vi "Fibonacci Sequence Custom Test.vi"(3 "Error In":errorcluster, 4 "Solution VI":path, 5 "User VI":path) -> (0 "Error Out":errorcluster, 2 "Results":T1={"Id"="", "Score"={"Status"=enum."Passed", "cpu_time"=-1, "max_memory"=-1, "style_score"=-1, "score0"="", "score1"="", "score2"="", "score3"="", "score4"="", "score5"=""}})   [LabVIEW 2013]
doc: "This VI is a template for a custom users test. The User VI control will provide the absolute path to the VI to test. The solution VI control will provide the absolute path to the solution VI. The Results indicator should be populated with the results from testing the user submitted VI."
uses:
  <vilib>/LabVIEW Hacker/VIChallenge/Private/Grader/Type Defs/Grader Result.ctl
  <vilib>/LabVIEW Hacker/VIChallenge/Private/Type Defs/Database/Score.ctl
  <vilib>/LabVIEW Hacker/VIChallenge/Private/Grader/Type Defs/UTF Status.ctl
  <vilib>/LabVIEW Hacker/VIChallenge/VIChallenge.lvlib
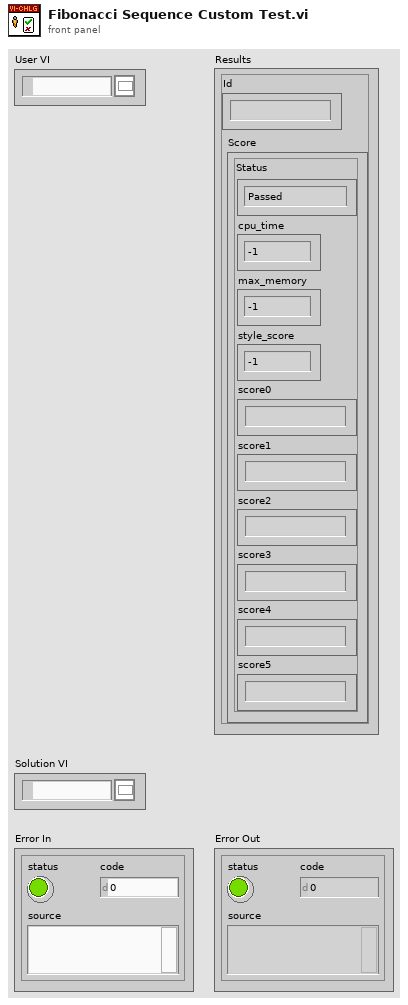
[diagram p1: front panel]
types:
  T1 = typedef "VIChallenge.lvlib/Grader Result.ctl" = cluster{"Id":string, "Score":T2}
  T2 = typedef "VIChallenge.lvlib/Score.ctl" = cluster{"Status":T3, "cpu_time":i32, "max_memory":i32, "style_score":i32, "score0":string, "score1":string, "score2":string, "score3":string, "score4":string, "score5":string}
  T3 = typedef "VIChallenge.lvlib/UTF Status.ctl" = enum16{"Null", "Passed", "Failed", "Error", "Skipped", "Not Processed"}
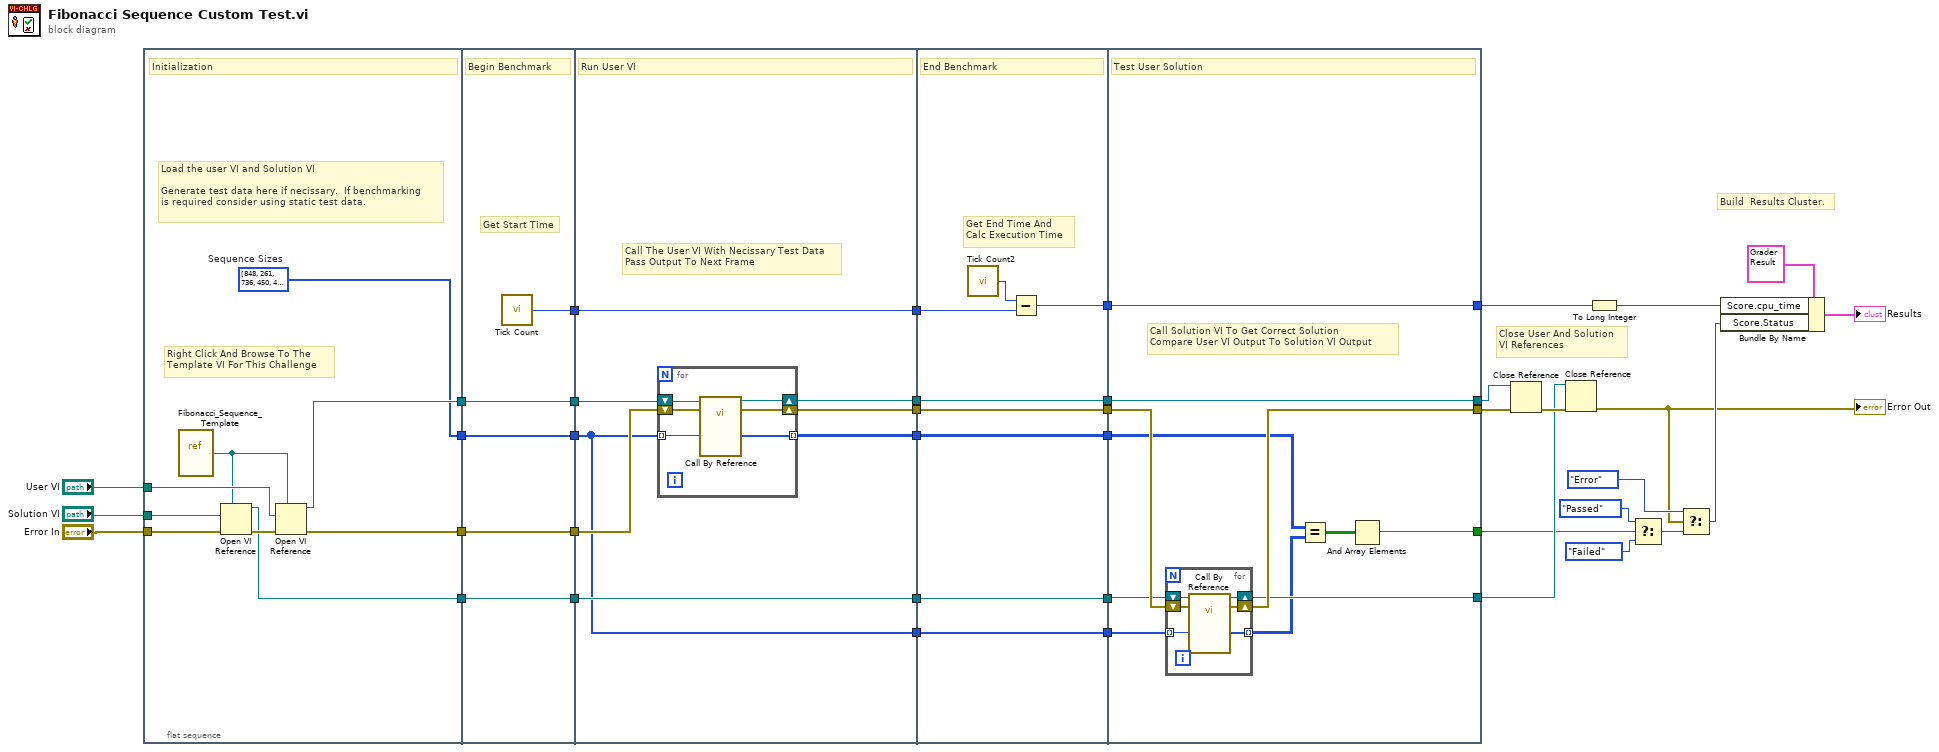
[diagram p0: block diagram]
diagram:
  # "Build  Results Cluster."
  # "Close User And Solution\nVI References"
  n1 = flat-sequence {
    tunnel: "User VI" -> [w48]
    tunnel: "Solution VI" -> [w47]
    tunnel: "Error In" -> [w45]
    tunnel: [w43] -> w36
    tunnel: [w42] -> w33
    tunnel: [w41] -> w31
    tunnel: [w40] -> w5
    tunnel: w36 -> [w53]
    tunnel: [w53] -> w35
    tunnel: [w52] -> w34
    tunnel: w33 -> [w52]
    tunnel: [w51] -> w32
    tunnel: w31 -> [w51]
    tunnel: [w50] -> w28
    tunnel: [w49] -> w6
    tunnel: w5 -> [w49]
    tunnel: w35 -> [w61]
    tunnel: w34 -> [w56]
    tunnel: w32 -> [w58]
    tunnel: [w60] -> w30
    tunnel: [w59] -> w29
    tunnel: w28 -> [w59]
    tunnel: [w58] -> w27
    tunnel: [w57] -> w24
    tunnel: w6 -> [w54]
    tunnel: [w55] -> w4
    tunnel: [w54] -> w2
    tunnel: w30 -> [w75]
    tunnel: w29 -> [w73]
    tunnel: w27 -> [w71]
    tunnel: [w75] -> w26
    tunnel: [w72] -> w25
    tunnel: w24 -> [w72]
    tunnel: [w71] -> w23
    tunnel: [w70] -> w16
    tunnel: w4 -> [w69]
    tunnel: [w69] -> w3
    tunnel: w2 -> [w68]
    tunnel: [w68] -> w1
    tunnel: w26 -> [w86]
    tunnel: [w85] -> w21
    tunnel: w25 -> [w84]
    tunnel: w23 -> [w81]
    tunnel: [w84] -> w22
    tunnel: [w83] -> w19
    tunnel: [w77] -> w10
    tunnel: [w82] -> w8
    tunnel: w16 -> [w82]
    tunnel: w3 -> [w79]
    tunnel: w1 -> [w76]
    frame #0 {
      w40 = i32[] [848, 261, 736, 450, 49, 224, 115, 680, 362, 624, 388, 820, 380, 134, 918, 80, 325, 741, 294, 696, 691, 389, 915, 94, 83, 534, 690, 884, 357, 231, 350, 306, 397, 577, 143, 331, 674, 651, 1, 955, 283, 492, 300, 331, 708, 110, 471, 604, 662, 688, 974, 81, 248, 860, 939, 728, 688, 739, 914, 177, 478, 553, 362, 47, 974, 305, 23, 21, 961, 618, 48, 320, 824, 858, 708, 83, 455, 633, 566, 303, 59, 686, 446, 422, 553, 816, 890, 2, 124, 380, 763, 747, 589, 93, 187, 708, 580, 173, 140, 759, 875, 436, 81, 583, 744, 843, 55, 23, 506, 335, 786, 137, 961, 736, 735, 404, 389, 322, 516, 500, 871, 607, 169, 214, 714, 459, 981, 620, 127, 889, 996, 708, 646, 29, 17, 401, 67, 538, 594, 639, 844, 321, 534, 599, 949, 132, 959, 525, 926, 960, 244, 913, 765, 714, 731, 554, 404, 451, 552, 639, 884, 506, 368, 394, 643, 586, 679, 689, 152, 774, 886, 928, 397, 633, 717, 929, 746, 21, 458, 364, 305, 218, 804, 475, 133, 567, 281, 12, 347, 932, 314, 835, 578, 181, 993, 288, 712, 262, 260, 91, 964, 436, 327, 78, 878, 660, 65, 334, 547, 455, 778, 594, 121, 44, 489, 594, 881, 98, 813, 344, 90, 360, 406, 840, 774, 262, 998, 166, 46, 997, 788, 862, 536, 417, 925, 762, 322, 598, 370, 909, 748, 627, 584, 320, 282, 604, 44, 710, 497, 951, 335, 283, 91, 467, 946, 286, 489, 482, 87, 572, 862, 986, 787, 68, 195, 928, 903, 904, 126, 315, 95, 514, 475, 508, 853, 889, 676, 678, 847, 157, 343, 368, 75, 163, 836, 3, 966, 743, 798, 794, 237, 376, 413, 65, 582, 245, 774, 480, 829, 614, 686, 122, 514, 932, 846, 794, 954, 919, 415, 973, 23, 812, 378, 892, 469, 770, 425, 619, 816, 806, 624, 930, 396, 924, 740, 375, 364, 624, 699, 2, 185, 252, 89, 251, 824, 889, 358, 576, 761, 308, 923, 706, 486, 608, 91, 184, 203, 396, 828, 131, 551, 331, 927, 347, 107, 109, 761, 87, 604, 488, 493, 846, 311, 631, 718, 289, 455, 96, 6, 201, 112, 115, 41, 144, 712, 178, 234, 10, 243, 314, 219, 630, 933, 189, 994, 272, 630, 689, 786, 645, 666, 962, 473, 347, 638, 288, 419, 479, 61, 892, 642, 116, 159, 121, 959, 127, 689, 78, 442, 139, 225, 401, 885, 423, 301, 523, 728, 503, 196, 240, 706, 88, 328, 817, 945, 290, 424, 898, 100, 923, 563, 494, 988, 623, 397, 721, 670, 5, 211, 665, 13, 983, 56, 546, 475, 834, 15, 267, 949, 679, 62, 883, 726, 338, 746, 647, 180, 663, 225, 811, 859, 193, 194, 622, 754, 36, 699, 553, 75, 272, 335, 411, 549, 283, 118, 596, 976, 703, 441, 757, 926, 643, 756, 972, 890, 809, 436, 888, 959, 628, 728, 440, 109, 936, 547, 85, 481, 662, 473, 998, 142, 523, 970, 102, 646, 409, 813, 527, 60, 964, 731, 626, 129, 447, 710, 341, 910, 783, 339, 323, 585, 789, 799, 348, 594, 900, 60, 187, 501, 465, 62, 342, 299, 766, 881, 852, 242, 797, 750, 195, 47, 147, 305, 346, 164, 729, 603, 95, 221, 599, 936, 835, 98, 563, 343, 600, 448, 901, 261, 506, 895, 123, 618, 247, 723, 111, 33, 622, 791, 146, 844, 893, 264, 193, 140, 812, 415, 964, 139, 451, 646, 421, 102, 219, 841, 462, 558, 685, 158, 566, 78, 620, 638, 871, 637, 255, 838, 673, 432, 706, 240, 394, 919, 183, 151, 623, 472, 154, 598, 386, 985, 310, 44, 434, 942, 798, 128, 603, 262, 830, 412, 468, 638, 461, 970, 391, 78, 305, 91, 931, 936, 536, 401, 833, 166, 652, 115, 107, 146, 662, 259, 508, 298, 100, 895, 783, 482, 689, 71, 542, 324, 325, 967, 615, 582, 917, 651, 753, 575, 395, 517, 391, 912, 482, 970, 847, 337, 148, 567, 853, 763, 815, 510, 317, 576, 546, 385, 843, 683, 614, 828, 683, 350, 881, 604, 470, 521, 834, 619, 198, 719, 493, 870, 299, 89, 868, 360, 825, 583, 845, 636, 800, 387, 697, 277, 41, 108, 542, 250, 72, 772, 558, 586, 116, 253, 576, 407, 9, 762, 737, 551, 902, 595, 757, 422, 749, 63, 247, 6, 860, 221, 691, 199, 470, 459, 119, 202, 214, 626, 574, 99, 331, 231, 838, 933, 251, 629, 643, 57, 200, 368, 858, 551, 181, 308, 428, 654, 482, 434, 209, 189, 824, 611, 981, 166, 259, 750, 298, 415, 582, 736, 14, 783, 840, 240, 999, 364, 850, 15, 108, 561, 200, 33, 736, 873, 429, 990, 447, 583, 935, 617, 989, 242, 693, 950, 379, 859, 740, 503, 546, 586, 837, 172, 264, 709, 711, 159, 187, 136, 633, 432, 985, 157, 144, 839, 491, 746, 741, 457, 318, 386, 456, 129, 64, 661, 262, 409, 472, 577, 720, 610, 99, 166, 181, 952, 359, 128, 375, 239, 811, 732, 260, 576, 57, 173, 334, 611, 583, 171, 388, 318, 462, 594, 27, 662, 567, 844, 850, 847, 301, 486, 99, 579, 296, 865, 713, 153, 480, 724, 632, 613, 807, 88, 963, 833, 129, 314, 592, 102, 368, 541, 329, 39, 939, 506, 862, 762, 262, 169, 550, 908, 927, 763, 179, 564, 182, 718, 687, 126, 835, 606, 37, 598, 308, 819, 697, 488, 36, 419, 912, 473, 453, 231, 475, 566, 651, 443, 162, 286, 935, 589, 930, 905, 615, 67, 584, 279, 570, 73, 910, 739, 430, 978, 484, 789, 808, 786, 5, 840, 566, 639, 300, 661, 526, 429, 209, 179, 371, 372, 568, 38, 97, 840, 843, 898, 344, 820, 882, 724, 348, 423, 102, 808, 382, 953, 339, 721, 687, 426, 508, 258, 477, 119, 980, 920, 833, 309, 426, 361, 462, 767, 197, 748, 164, 557, 872, 447, 153, 224, 761, 580, 807, 795, 756, 459, 723, 204, 614, 773, 787]  # Sequence Sizes
      # "Load the user VI and Solution VI\n\nGenerate test data here if necissary.  If benchmarking \nis required consider using static test data."
      # "Right Click And Browse To The \nTemplate VI For This Challenge"
      # "Initialization"
      n2 = vi-ref <vilib>:"Fibonacci_Sequence_Template.vi"() -> (w46:refnum<vi>)
      n3 = Open VI Reference(type specifier VI Refnum (for type only)=w46, vi path=w47, error in (no error)=w45) -> (vi reference=w41:refnum<vi>, error out=w44:errorcluster)  [unwired: 3 in]
      n4 = Open VI Reference(type specifier VI Refnum (for type only)=w46, vi path=w48, error in (no error)=w44) -> (vi reference=w42:refnum<vi>, error out=w43:errorcluster)  [unwired: 3 in]
    }
    frame #1 {
      # "Get Start Time"
      # "Begin Benchmark"
      n5 = call "Tick Count"() -> ("Tick Count(uSec)"=w50:u32)
    }
    frame #2 {
      # "Call The User VI With Necissary Test Data\nPass Output To Next Frame"
      # "Run User VI"
      n6 = for {
        tunnel: w54 -> [w63] mode=indexing
        shift-right: [w66] -> w60
        shift-left: w61 -> [w67]
        tunnel: [w62] -> w55 mode=indexing
        shift-right: [w65] -> w57
        shift-left: w56 -> [w64]
        n7 = call-by-ref "?"(reference=w64, error in=w67, "Sequence Size"=w63) -> (reference out=w65:refnum<vi>, error out=w66:errorcluster, "Fibonacci Sequence"=w62:i32[])  [unwired: 4 in]
      }
    }
    frame #3 {
      # "Get End Time And \nCalc Execution Time"
      # "End Benchmark"
      n8 = call "Tick Count2"() -> ("Tick Count(uSec)"=w74:u32)
      n9 = Subtract(x=w74, y=w73) -> (x-y=w70:u32)
    }
    frame #4 {
      # "Call Solution VI To Get Correct Solution\nCompare User VI Output To Solution VI Output"
      # "Test User Solution"
      n10 = for {
        shift-right: [w90] -> w83
        shift-left: w81 -> [w89]
        tunnel: [w88] -> w80 mode=indexing
        shift-right: [w91] -> w85
        shift-left: w86 -> [w92]
        tunnel: w76 -> [w87] mode=indexing
        n11 = call-by-ref "?"(reference=w89, error in=w92, "Sequence Size"=w87) -> (reference out=w90:refnum<vi>, error out=w91:errorcluster, "Fibonacci Sequence"=w88:i32[])  [unwired: 4 in]
      }
      n12 = Equal?(x=w79, y=w80) -> (x = y?=w78:bool[][])
      n13 = And Array Elements(Boolean array=w78) -> (logical AND=w77:bool)
    }
  }
  n14 = Close Reference(reference=w22, error in (no error)=w21) -> (error out=w20:errorcluster)
  n15 = Close Reference(reference=w19, error in (no error)=w20) -> (error out=w9:errorcluster)
  "Error Out" <- w9
  n16 = To Long Integer(number=w8) -> (32bit integer=w7:i32)
  n17 = Select(t=UTF_Status."Passed" ("Score.Status"), s=w10, f=UTF_Status."Failed" ("Score.Status")) -> (s? t:f=w13:T3)
  n18 = Select(t=UTF_Status."Error", s=w9, f=w13) -> (s? t:f=w11:T3)
  n19 = Bundle By Name(cluster=T1 {"Id"="", "Score"={"Status"=enum."Passed", "cpu_time"=-1, "max_memory"=-1, "style_score"=-1, "score0"="", "score1"="", "score2"="", "score3"="", "score4"="", "score5"=""}} ("Results"), "Score.cpu_time"=w7, "Score.Status"=w11) -> (→"Results":T1)
